vi "Simple UDP - Receiver.vi"() -> ()   [LabVIEW 2020]
doc: "UDP协议与TCP的区别在于UDP不包括发送数据包信息的错误检查，因此无法保证接收端是否已接收所发数据。\n\nUDP可用于“广播”数据至整个网络，只需指定可包括全部的IP地址(255.255.255.255)以便发送信息至整个网络。 由于路由器或其他网络硬件通常拒绝转发超过一定点的数据，在实际应用中广播范围可能存在限制。"
panel:
  out "元素":i32[][](array[numeric])
  in  "停止 2":bool
  out "波形图表 5":i32[](graph)
  # "概述：演示使用UDP函数通过UDP连接接收数据。\n操作步骤：\n1.确保已运行Simple UDP - Sender.vi。\n2.运行VI。\n3.单击停止按钮停止VI。"
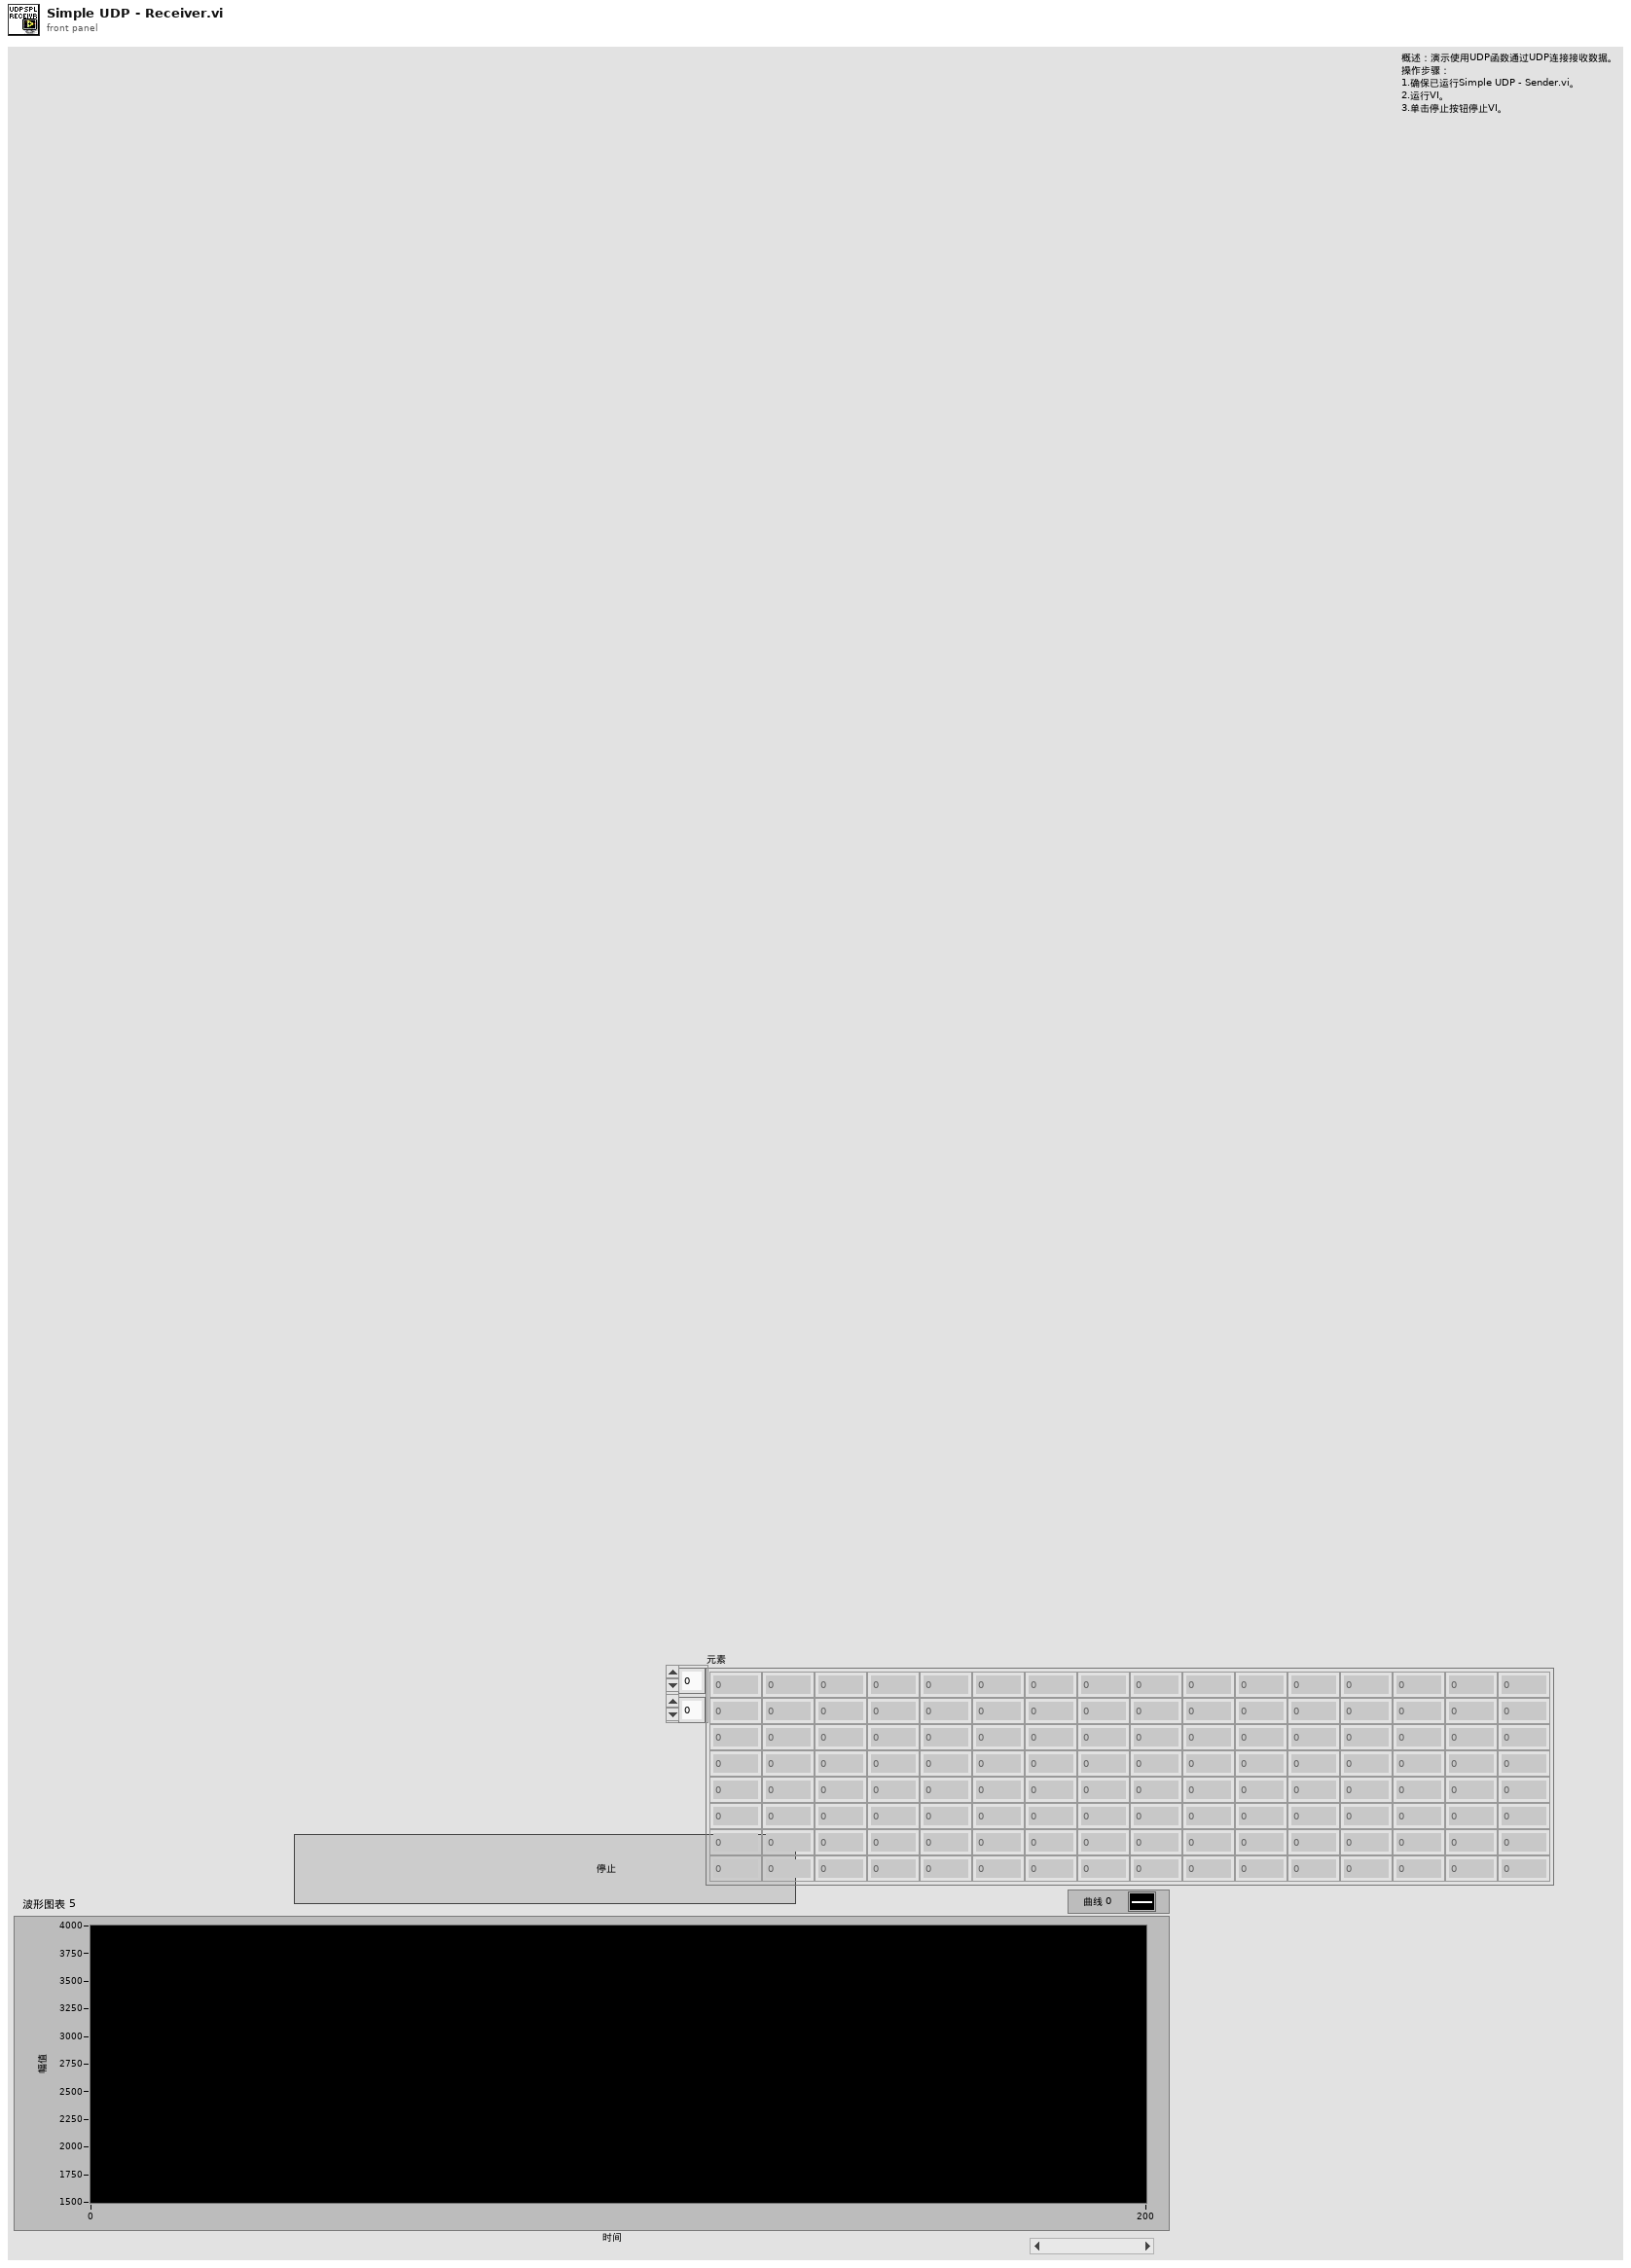
[diagram p1: front panel]
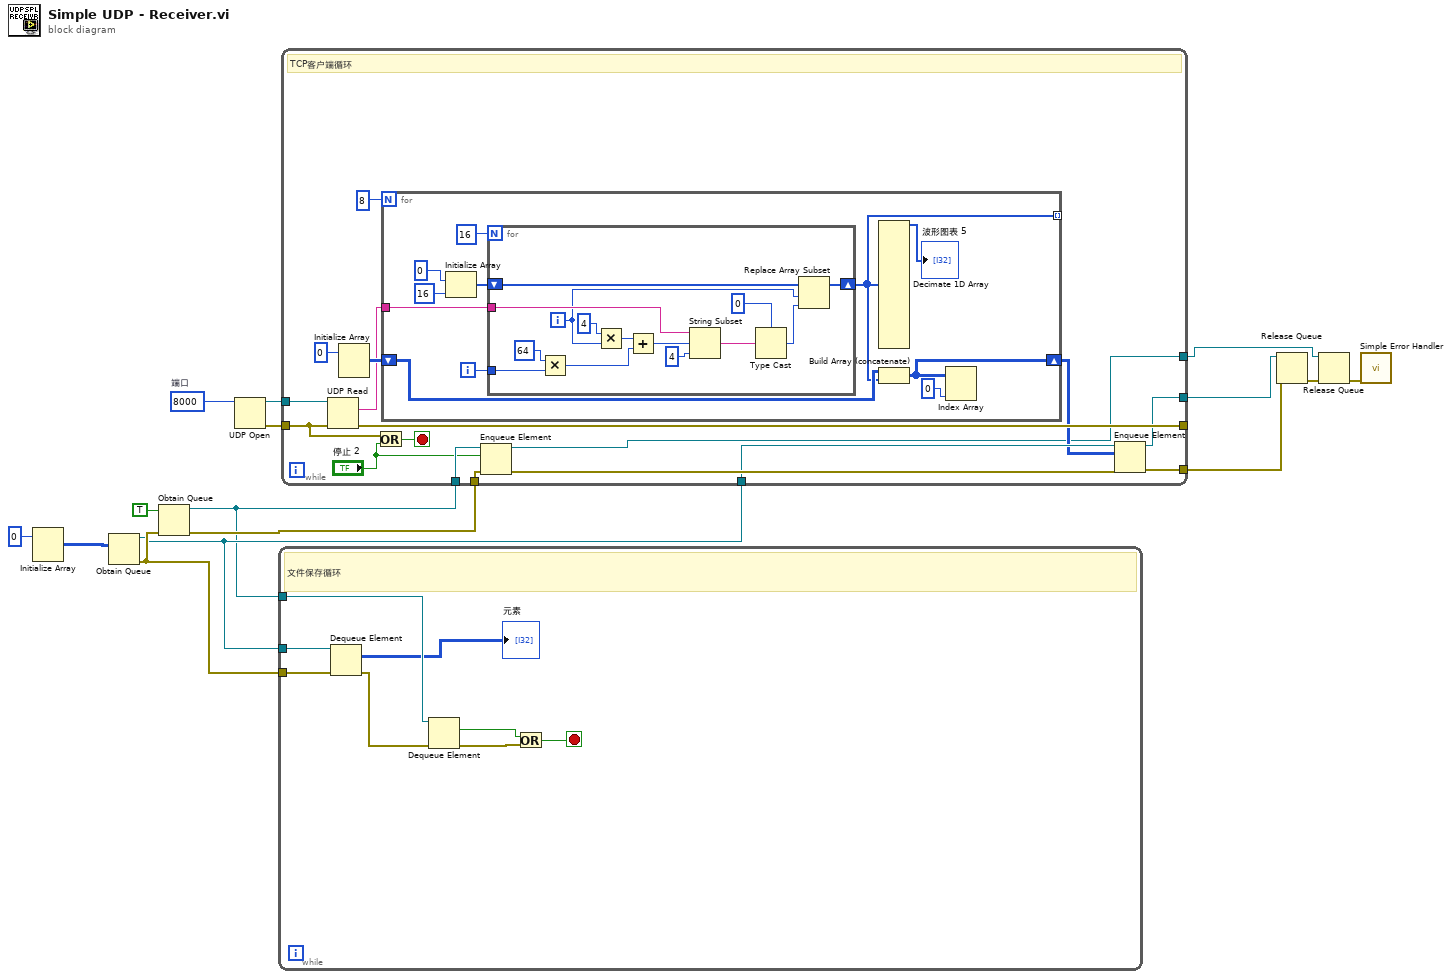
[diagram p0: block diagram]
diagram:
  w12 = u16 8000  # 端口
  n1 = Initialize Array(0) -> (w10:i32[][])  [unwired: 2 in]
  n2 = Obtain Queue(element data type=w10) -> (queue out=w2:refnum<queue>, error out=w3:errorcluster)  [unwired: 4 in, 1 out]
  n3 = Obtain Queue(element data type=TRUE, error in (no error)=w3) -> (queue out=w1:refnum<queue>, error out=w9:errorcluster)  [unwired: 3 in, 1 out]
  n4 = UDP Open(11:w12) -> (port=w14:refnum<k16>, 0:w13:errorcluster)  [unwired: 4 in, 1 out]
  n5 = while {
    tunnel: w3 -> [w23]
    tunnel: w2 -> [w21]
    tunnel: w1 -> [w19]
    stop <- w22 stop-if-true
    # "文件保存循环"
    n6 = Dequeue Element(queue=w21, error in (no error)=w23) -> (element=→"元素":i32[][], error out=w20:errorcluster)  [unwired: 1 in, 2 out]
    n7 = Dequeue Element(queue=w19, error in (no error)=w20) -> (element=w18:bool, error out=w17:errorcluster)  [unwired: 1 in, 2 out]
    n8 = Or(x=w18, y=w17) -> (x .or. y?=w22:bool)
  }
  n9 = while {
    tunnel: w13 -> [w35]
    tunnel: w14 -> [w34]
    tunnel: [w36] -> _
    tunnel: w1 -> [w32]
    tunnel: w9 -> [w30]
    tunnel: w2 -> [w28]
    tunnel: [w26] -> w6
    tunnel: [w25] -> w5
    tunnel: [w24] -> w4
    stop <- w38 stop-if-true
    # "TCP客户端循环"
    n10 = UDP Read(connection ID=w34, 8:w35) -> (data out=w37:string, error out=w36:errorcluster)  [unwired: 1 in, 4 out]
    n11 = Initialize Array(0) -> (w39:i32[][])  [unwired: 2 in]
    n12 = Or(x=w35, y="停止 2") -> (x .or. y?=w38:bool)
    n13 = for {
      N: u16 8 -> [_]
      tunnel: w37 -> [w51]
      shift-right: [w44] -> w27
      shift-left: w39 -> [w45]
      tunnel: [w41] -> _ mode=indexing
      i -> [w46]
      n14 = Initialize Array(0, 16) -> (w47:i32[])
      n15 = for {
        N: i8 16 -> [_]
        tunnel: w51 -> [w63]
        tunnel: w46 -> [w59]
        shift-right: [w52] -> w41
        shift-left: w47 -> [w53]
        i -> [w54]
        n16 = Multiply(x=i8 64, y=w59) -> (x*y=w58:i32)
        n17 = Multiply(x=i8 4, y=w54) -> (x*y=w56:i32)
        n18 = Add(x=w56, y=w58) -> (x+y=w57:i32)
        n19 = String Subset(string=w63, offset (0)=w57, length (rest)=i8 4) -> (substring=w65:string)
        n20 = Type Cast(type=0, x=w65) -> (*(type *) &x=w55:i32)
        n21 = Replace Array Subset(array=w53, new element=w55, index=w54) -> (w52:i32[])
      }
      n22 = Decimate 1D Array(w41) -> (→"波形图表 5":i32[])  [unwired: 15 out]
      n23 = Build Array (concatenate)(w45, w41) -> (w44:i32[][])
      n24 = Index Array(array=w44, index (col)=0) -> ()  [unwired: 1 in, 1 out]
    }
    n25 = Enqueue Element(queue=w32, element="停止 2", error in (no error)=w30) -> (queue out=w24:refnum<queue>, error out=w29:errorcluster)  [unwired: 1 in, 1 out]
    n26 = Enqueue Element(queue=w28, element=w27, error in (no error)=w29) -> (queue out=w25:refnum<queue>, error out=w26:errorcluster)  [unwired: 1 in, 1 out]
  }
  n27 = Release Queue(queue=w5, error in (no error)=w6) -> (error out=w8:errorcluster)  [unwired: 1 in, 2 out]
  n28 = Release Queue(queue=w4, error in (no error)=w8) -> (error out=w7:errorcluster)  [unwired: 1 in, 2 out]
  n29 = call <vilib>:"Simple Error Handler.vi"("error in (no error)"=w7) -> ()  [unwired: 4 in, 5 out]
